vi "Get specification uncertainty.vi"(8 "error in (no error)":errorcluster, 10 "Limit selection":u16(ring) items=["Low limit", "High limit"], 11 "VISA resource name":refnum<visa-resource-name>) -> (0 "error out":errorcluster, 1 "24 hour string":string, 2 "24 hours":dbl, 3 "VISA resource name out":refnum<visa-resource-name>, 4 "1 year string":string, 5 "90 days string":string, 6 "1 year":dbl, 7 "90 days":dbl)   [LabVIEW 2012, in "Datron D4xxx.lvlib"]
doc: "This VI returns specification uncertainties added to current value (low or high value limit)."
uses:
  Datron D4xxx.lvlib
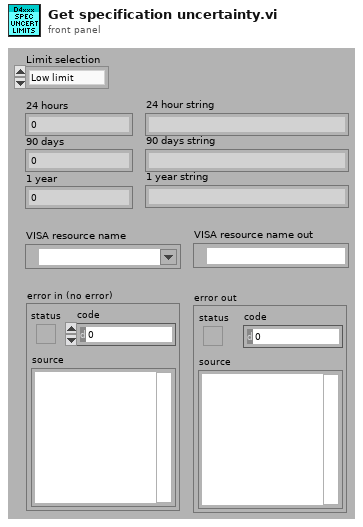
[diagram p1: front panel]
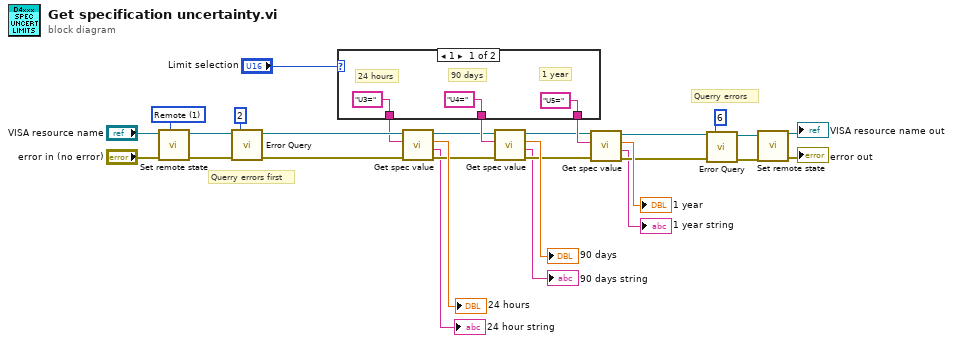
[diagram p0: block diagram]
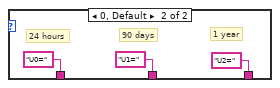
[diagram p2: hidden frame]
diagram:
  w27 = u16 1 items=["Local", "Remote", "Default"] ("Remote state")
  # "Querry errors"
  # "Querry errors first"
  n1 = call "Set remote state.vi"("error in"="error in (no error)", "Remote state"=w27, "VISA resource name"="VISA resource name") -> ("error out"=w24:errorcluster, "VISA resource name out"=w23:refnum<visa-resource-name>)  [unwired: 7 in]
  n2 = call "Error Query.vi"("error in (no error)"=w24, "Check cycles (11)"=2, "VISA resource name"=w23) -> ("error out"=w21:errorcluster, "VISA resource name out"=w20:refnum<visa-resource-name>)  [unwired: 5 in, 2 out]
  n3 = case shown="1" "Limit selection" {
    tunnel: ["U3=" ("write buffer") "U0=" ("write buffer")] -> w11
    tunnel: ["U4=" ("write buffer") "U1=" ("write buffer")] -> w10
    tunnel: ["U5=" ("write buffer") "U2=" ("write buffer")] -> w9
    frame 1 {
      # "1 year"
      # "90 days"
      # "24 hours"
    }
    frame 0, Default {
      # "1 year"
      # "90 days"
      # "24 hours"
    }
  }
  n4 = call "Get spec value.vi"("error in (no error)"=w21, "Command string"=w11, "VISA resource name"=w20) -> ("error out"=w8:errorcluster, "Value string"=→"24 hour string":string, "Value"=→"24 hours":dbl, "VISA resource name out"=w6:refnum<visa-resource-name>)  [unwired: 5 in]
  n5 = call "Get spec value.vi"("error in (no error)"=w8, "Command string"=w10, "VISA resource name"=w6) -> ("error out"=w7:errorcluster, "Value string"=→"90 days string":string, "Value"=→"90 days":dbl, "VISA resource name out"=w5:refnum<visa-resource-name>)  [unwired: 5 in]
  n6 = call "Get spec value.vi"("error in (no error)"=w7, "Command string"=w9, "VISA resource name"=w5) -> ("error out"=w16:errorcluster, "Value string"=→"1 year string":string, "Value"=→"1 year":dbl, "VISA resource name out"=w15:refnum<visa-resource-name>)  [unwired: 5 in]
  n7 = call "Error Query.vi"("error in (no error)"=w16, "Check cycles (11)"=6, "VISA resource name"=w15) -> ("error out"=w12:errorcluster, "VISA resource name out"=w13:refnum<visa-resource-name>)  [unwired: 5 in, 2 out]
  n8 = call "Set remote state.vi"("error in"=w12, "VISA resource name"=w13) -> ("error out"=→"error out":errorcluster, "VISA resource name out"=→"VISA resource name out":refnum<visa-resource-name>)  [unwired: 8 in]
